vi "NewLogToSpreadsheet.vi"() -> ()   [LabVIEW 2012]
doc: "Reads new (11-1-2012+) style logs and displays the data in a human-understandable format."
uses:
  2-Think/2 Typedefs/UTM Circle.ctl
  2-Think/2 Typedefs/UTM Location.ctl
  <vilib>/Utility/file.llb/Write To Spreadsheet File (DBL).vi
panel:
  in  "Array":string[](array[string])=["RobotLocation", "RobotHeading", "RobotVelocity", "RobotPitch", "RobotRoll", "BatteryVoltage", "ApparentWindDirection", "ApparentWindSpeed", "Rudder", "Sail", "GoodnessFunctions", "NoSailZones", "Waypoint#", "WaypointTolerance", "WaypointCoordinates", "OverrideRudder", "OverrideSail"]
  out "Processing File....":path
  in  "Stop early":bool
  out "Percent Complete":u8(slide) scale=0.0..100.0
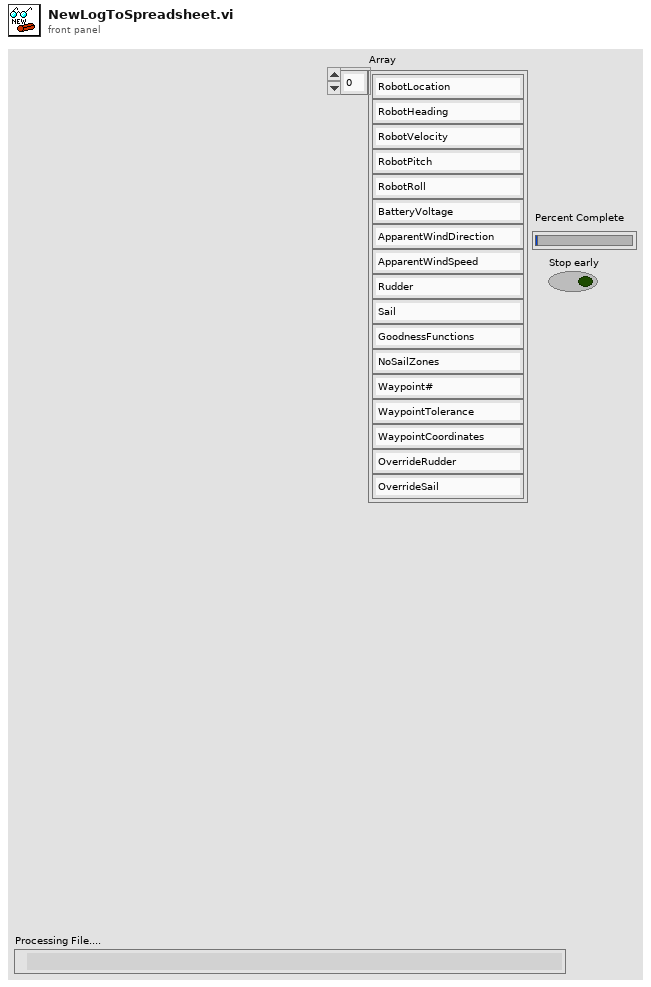
[diagram p1: front panel]
types:
  T1 = typedef "UTM Circle.ctl" = cluster{"UTM Zone":dbl, "Hemisphere":enum16{"North", "South"}, "East":dbl, "North":dbl, "Radius":dbl}
  T2 = typedef "UTM Location.ctl" = cluster{"UTM Zone":dbl, "Hemisphere":enum16{"North", "South"}, "East":dbl, "North":dbl}
  T3 = cluster{"RobotHeading":dbl, "RobotSpeed":dbl, "RobotPitch":dbl, "RobotRoll":dbl, "BatteryVoltage":dbl, "ApparentWindDirection":dbl, "ApparentWindSpeed":dbl, "Rudder":dbl, "Sail":dbl, "Waypoint#":dbl, "WaypointTolerance":dbl, "GoodnessFunctions":string, "OverrideRudder":bool, "OverrideSail":bool, "Global No Sail Circles":T1[], "Robot Location":T2, "WaypointCoordinates":T2}
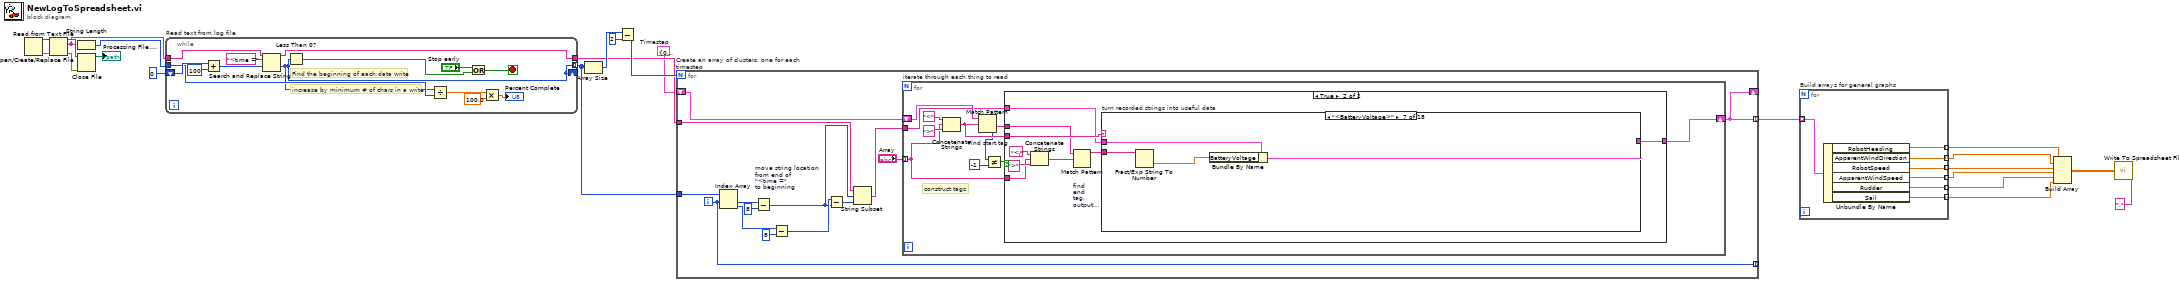
[diagram p0: block diagram]
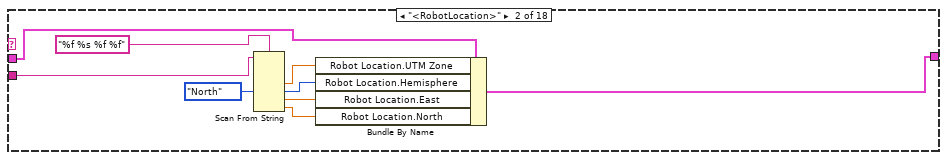
[diagram p4: hidden frame]
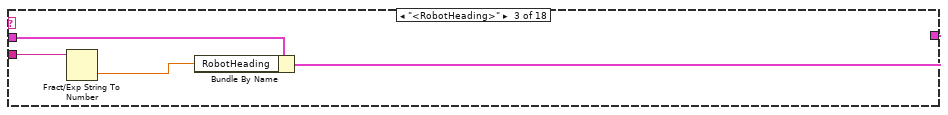
[diagram p5: hidden frame]
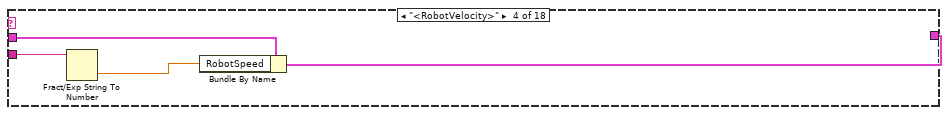
[diagram p6: hidden frame]
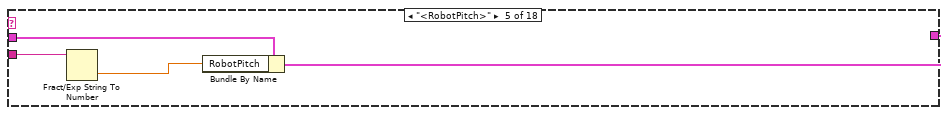
[diagram p7: hidden frame]
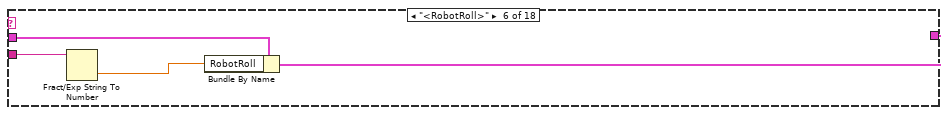
[diagram p8: hidden frame]
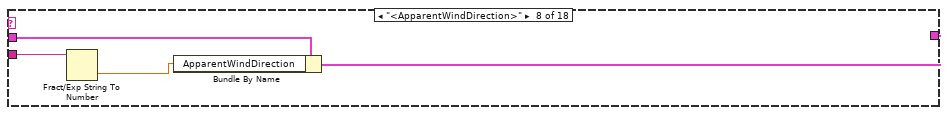
[diagram p9: hidden frame]
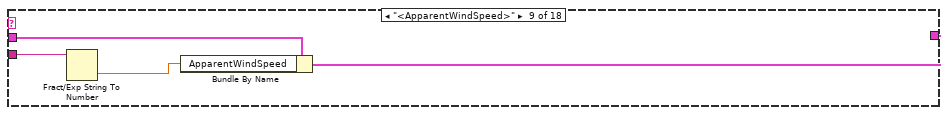
[diagram p10: hidden frame]
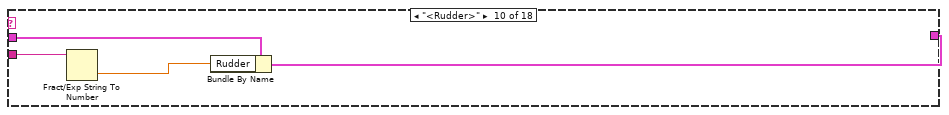
[diagram p11: hidden frame]
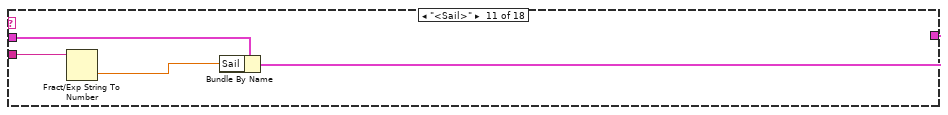
[diagram p12: hidden frame]
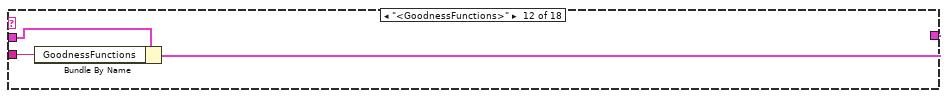
[diagram p13: hidden frame]
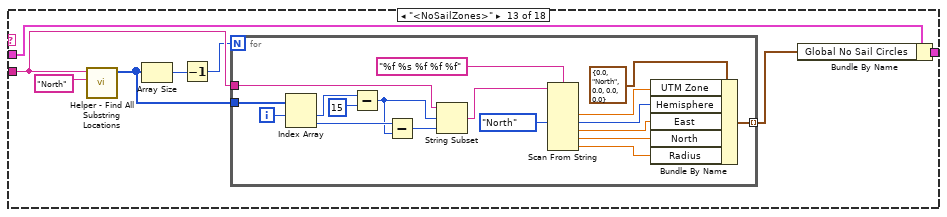
[diagram p14: hidden frame]
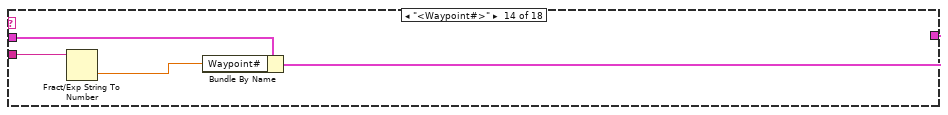
[diagram p15: hidden frame]
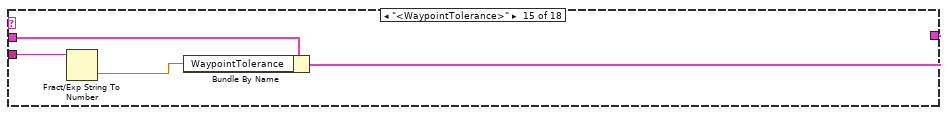
[diagram p16: hidden frame]
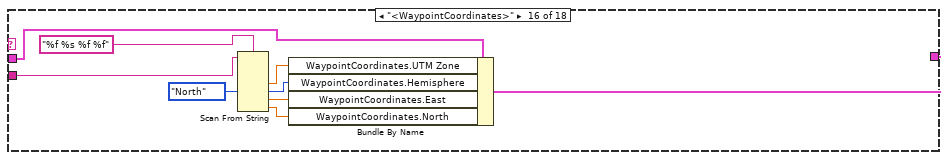
[diagram p17: hidden frame]
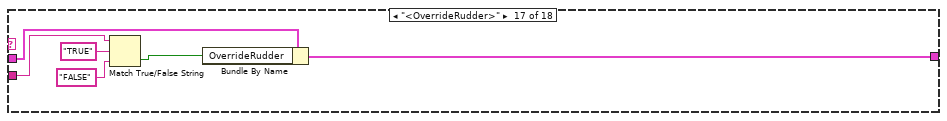
[diagram p18: hidden frame]
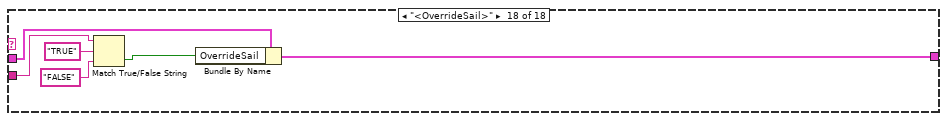
[diagram p19: hidden frame]
diagram:
  w10 = T3 {"RobotHeading"=0.0, "RobotSpeed"=0.0, "RobotPitch"=0.0, "RobotRoll"=0.0, "BatteryVoltage"=0.0, "ApparentWindDirection"=0.0, "ApparentWindSpeed"=0.0, "Rudder"=0.0, "Sail"=0.0, "Waypoint#"=0.0, "WaypointTolerance"=0.0, "GoodnessFunctions"="", "OverrideRudder"=FALSE, "OverrideSail"=FALSE, "Global No Sail Circles"=[], "Robot Location"={"UTM Zone"=0.0, "Hemisphere"=enum."North", "East"=0.0, "North"=0.0}, "WaypointCoordinates"={"UTM Zone"=0.0, "Hemisphere"=enum."North", "East"=0.0, "North"=0.0}}  # Timestep
  n1 = Open/Create/Replace File() -> (refnum out=w23:refnum<file>, error out=w19:errorcluster)  [unwired: 6 in, 1 out]
  n2 = Read from Text File(file (use dialog)=w23, error in=w19) -> (refnum out=w20:refnum<file>, text=w17:string, error out=w21:errorcluster)  [unwired: 2 in, 1 out]
  n3 = String Length(string=w17) -> (length=w16:i32)
  n4 = Close File(refnum=w20, error in=w21) -> (path=→"Processing File....":path)  [unwired: 1 out]
  n5 = while "Read text from log file" {
    tunnel: w17 -> [w27]
    shift-right: [w25] -> _
    shift-left: 0 ("offset past replacement") -> [w37]
    tunnel: [w26] -> w11
    tunnel: [w25] -> w12 mode=indexing
    tunnel: w16 -> [w29]
    stop <- w35 stop-if-true
    # "increase by minimum # of chars in a write"
    # "Find the beginning of each data write"
    n6 = Add(x=w37, y=100) -> (x+y=w28:i32)
    n7 = Search and Replace String(input string=w27, search string="<time =", offset=w28) -> (result string=w26:string, offset past replacement=w25:i32)  [unwired: 5 in, 2 out]
    n8 = Less Than 0?(x=w25) -> (x < 0?=w33:bool)
    n9 = Divide(x=w25, y=w29) -> (x/y=w32:dbl)
    n10 = Or(x="Stop early", y=w33) -> (x .or. y?=w35:bool)
    n11 = Multiply(x=w32, y=100.0) -> (x*y=→"Percent Complete":dbl)
  }
  n12 = Array Size(array=w12) -> (size(s)=w15:i32)
  n13 = Subtract(x=w15, y=2) -> (x-y=w13:i32)
  n14 = for "Create an array of clusters, one for each timestep" {
    N: w13 -> [_]
    tunnel: w12 -> [w51]
    tunnel: w11 -> [w46]
    tunnel: [w42] -> w9 mode=indexing
    shift-right: [w42] -> _
    shift-left: w10 -> [w41]
    tunnel: [w38] -> _ mode=indexing
    i -> [w38]
    n15 = Index Array(array=w51, index #1=w38) -> (element #1=w50:i32, element #2=w47:i32)  [unwired: 1 in]
    n16 = Subtract "move string location\nfrom end of \n\"<time =\"\nto beginning"(x=w50, y=8) -> (x-y=w39:i32)
    n17 = Subtract(x=w47, y=8) -> (x-y=w40:i32)
    n18 = Subtract(x=w40, y=w39) -> (x-y=w45:i32)
    n19 = String Subset(string=w46, offset (0)=w39, length (rest)=w45) -> (substring=w44:string)
    n20 = for "iterate through each thing to read" {
      tunnel: w44 -> [w61]
      tunnel: "Array" -> [w59] mode=indexing
      shift-right: [w57] -> w42
      shift-left: w41 -> [w55]
      # "construct tags"
      n21 = Concatenate Strings("<" ("string"), w59, ">" ("string")) -> (w60:string)
      n22 = Match Pattern "Find start tag"(string=w61, regular expression=w60) -> (after substring=w56:string, offset past match=w53:i32)  [unwired: 1 in, 2 out]
      n23 = Not Equal?(x=w53, y=-1) -> (x != y?=w54:bool)
      n24 = case shown="True" w54 {
        tunnel: w60 -> [_ w69]
        tunnel: w59 -> [_ w68]
        tunnel: [w63 w67] -> w57
        tunnel: w56 -> [_ w65]
        tunnel: w55 -> [w63 w64]
        frame False {
        }
        frame True {
          n25 = Concatenate Strings("</" ("string"), w68, ">" ("string")) -> (w70:string)
          n26 = Match Pattern "find\nend\ntag,\noutput\nbetween\ntags"(string=w65, regular expression=w70) -> (before substring=w66:string)  [unwired: 1 in, 3 out]
          n27 = case "turn recorded strings into useful data" shown="\"<BatteryVoltage>\"" w69 {
            tunnel: w66 -> [_ w76 w86 w89 w92 w97 w99 w103 w107 w111 w115 w120 w127 w149 w152 w156 w165 w171]
            tunnel: w64 -> [w73 w78 w85 w90 w93 w96 w101 w105 w109 w113 w117 w121 w126 w150 w154 w163 w168 w173]
            tunnel: [w73 w77 w83 w87 w91 w95 w100 w104 w108 w112 w116 w119 w124 w148 w153 w159 w166 w172] -> w67
            frame Default {
              # "hopefully never needs to be used"
            }
            frame "<RobotLocation>" {
              n28 = Scan From String(format string="%f %s %f %f", input string=w76, default 2=enum16{"North", "South"}."North" ("Robot Location.Hemisphere")) -> (output 1=w81:dbl, output 2=w74:enum16{"North", "South"}, output 3=w80:dbl, output 4=w79:dbl)  [unwired: 5 in, 3 out]
              n29 = Bundle By Name(cluster=w78, "Robot Location.UTM Zone"=w81, "Robot Location.Hemisphere"=w74, "Robot Location.East"=w80, "Robot Location.North"=w79) -> (w77:T3)
            }
            frame "<RobotHeading>" {
              n30 = Fract/Exp String To Number(string=w86) -> (number=w84:dbl)  [unwired: 3 in, 1 out]
              n31 = Bundle By Name(cluster=w85, "RobotHeading"=w84) -> (w83:T3)
            }
            frame "<RobotVelocity>" {
              n32 = Fract/Exp String To Number(string=w89) -> (number=w88:dbl)  [unwired: 3 in, 1 out]
              n33 = Bundle By Name(cluster=w90, "RobotSpeed"=w88) -> (w87:T3)
            }
            frame "<RobotPitch>" {
              n34 = Fract/Exp String To Number(string=w92) -> (number=w94:dbl)  [unwired: 3 in, 1 out]
              n35 = Bundle By Name(cluster=w93, "RobotPitch"=w94) -> (w91:T3)
            }
            frame "<RobotRoll>" {
              n36 = Fract/Exp String To Number(string=w97) -> (number=w98:dbl)  [unwired: 3 in, 1 out]
              n37 = Bundle By Name(cluster=w96, "RobotRoll"=w98) -> (w95:T3)
            }
            frame "<BatteryVoltage>" {
              n38 = Fract/Exp String To Number(string=w99) -> (number=w102:dbl)  [unwired: 3 in, 1 out]
              n39 = Bundle By Name(cluster=w101, "BatteryVoltage"=w102) -> (w100:T3)
            }
            frame "<ApparentWindDirection>" {
              n40 = Fract/Exp String To Number(string=w103) -> (number=w106:dbl)  [unwired: 3 in, 1 out]
              n41 = Bundle By Name(cluster=w105, "ApparentWindDirection"=w106) -> (w104:T3)
            }
            frame "<ApparentWindSpeed>" {
              n42 = Fract/Exp String To Number(string=w107) -> (number=w110:dbl)  [unwired: 3 in, 1 out]
              n43 = Bundle By Name(cluster=w109, "ApparentWindSpeed"=w110) -> (w108:T3)
            }
            frame "<Rudder>" {
              n44 = Fract/Exp String To Number(string=w111) -> (number=w114:dbl)  [unwired: 3 in, 1 out]
              n45 = Bundle By Name(cluster=w113, "Rudder"=w114) -> (w112:T3)
            }
            frame "<Sail>" {
              n46 = Fract/Exp String To Number(string=w115) -> (number=w118:dbl)  [unwired: 3 in, 1 out]
              n47 = Bundle By Name(cluster=w117, "Sail"=w118) -> (w116:T3)
            }
            frame "<GoodnessFunctions>" {
              n48 = Bundle By Name(cluster=w121, "GoodnessFunctions"=w120) -> (w119:T3)
            }
            frame "<NoSailZones>" {
              n49 = call "Helper - Find All Substring Locations.vi"("search string"="North", "input string"=w127) -> ("Locations"=w128:i32[])  [unwired: 9 in]
              n50 = Array Size(array=w128) -> (size(s)=w122:i32)
              n51 = Decrement(x=w122) -> (x-1=w123:i32)
              n52 = for {
                N: w123 -> [_]
                tunnel: w128 -> [w147]
                tunnel: w127 -> [w144]
                tunnel: [w134] -> w125 mode=indexing
                i -> [w133]
                n53 = Index Array(array=w147, index #1=w133) -> (element #1=w132:i32, element #2=w131:i32)  [unwired: 1 in]
                n54 = Subtract(x=w132, y=15) -> (x-y=w130:i32)
                n55 = Subtract(x=w131, y=w130) -> (x-y=w145:i32)
                n56 = String Subset(string=w144, offset (0)=w130, length (rest)=w145) -> (substring=w143:string)
                n57 = Scan From String(format string="%f %s %f %f %f", input string=w143, default 2=enum16{"North", "South"}."North" ("Hemisphere")) -> (output 1=w140:dbl, output 2=w138:enum16{"North", "South"}, output 3=w137:dbl, output 4=w136:dbl, output 5=w135:dbl)  [unwired: 6 in, 3 out]
                n58 = Bundle By Name(cluster=T1 {"UTM Zone"=0.0, "Hemisphere"=enum."North", "East"=0.0, "North"=0.0, "Radius"=0.0} ("UTM Location"), "UTM Zone"=w140, "Hemisphere"=w138, "East"=w137, "North"=w136, "Radius"=w135) -> (w134:T1)
              }
              n59 = Bundle By Name(cluster=w126, "Global No Sail Circles"=w125) -> (w124:T3)
            }
            frame "<Waypoint#>" {
              n60 = Fract/Exp String To Number(string=w149) -> (number=w151:dbl)  [unwired: 3 in, 1 out]
              n61 = Bundle By Name(cluster=w150, "Waypoint#"=w151) -> (w148:T3)
            }
            frame "<WaypointTolerance>" {
              n62 = Fract/Exp String To Number(string=w152) -> (number=w155:dbl)  [unwired: 3 in, 1 out]
              n63 = Bundle By Name(cluster=w154, "WaypointTolerance"=w155) -> (w153:T3)
            }
            frame "<WaypointCoordinates>" {
              n64 = Scan From String(format string="%f %s %f %f", input string=w156, default 2=enum16{"North", "South"}."North" ("WaypointCoordinates.Hemisphere")) -> (output 1=w162:dbl, output 2=w157:enum16{"North", "South"}, output 3=w161:dbl, output 4=w160:dbl)  [unwired: 5 in, 3 out]
              n65 = Bundle By Name(cluster=w163, "WaypointCoordinates.UTM Zone"=w162, "WaypointCoordinates.Hemisphere"=w157, "WaypointCoordinates.East"=w161, "WaypointCoordinates.North"=w160) -> (w159:T3)
            }
            frame "<OverrideRudder>" {
              n66 = Match True/False String(2:"FALSE" ("false string"), 3:"TRUE" ("true string"), 4:w165) -> (0:w167:bool)  [unwired: 1 out]
              n67 = Bundle By Name(cluster=w168, "OverrideRudder"=w167) -> (w166:T3)
            }
            frame "<OverrideSail>" {
              n68 = Match True/False String(2:"FALSE" ("false string"), 3:"TRUE" ("true string"), 4:w171) -> (0:w174:bool)  [unwired: 1 out]
              n69 = Bundle By Name(cluster=w173, "OverrideSail"=w174) -> (w172:T3)
            }
          }
        }
      }
    }
  }
  n70 = for "Build arrays for general graphs" {
    tunnel: w9 -> [w183] mode=indexing
    tunnel: [w182] -> w8 mode=indexing
    tunnel: [w181] -> w7 mode=indexing
    tunnel: [w180] -> w6 mode=indexing
    tunnel: [w179] -> w5 mode=indexing
    tunnel: [w178] -> w4 mode=indexing
    tunnel: [w177] -> w3 mode=indexing
    n71 = Unbundle By Name(w183) -> ("RobotHeading"=w182:dbl, "ApparentWindDirection"=w181:dbl, "RobotSpeed"=w180:dbl, "ApparentWindSpeed"=w179:dbl, "Rudder"=w178:dbl, "Sail"=w177:dbl)
  }
  n72 = Build Array(w8, w7, w6, w5, w4, w3) -> (w2:dbl[][])
  n73 = call-poly <vilib>:"Write To Spreadsheet File.vi"("delimiter (\\t)"="," ("delimiter (\\t)"), "2D data"=w2) -> ()  [unwired: 6 in, 1 out]
